vi "RecallState.vi"(8 "error in":errorcluster, 10 "File Name ()":string, 11 "C4209 PNA.lvclass 2":refnum<class "C4209 PNA.lvclass">) -> (0 "error out":errorcluster, 3 "C4209 PNA.lvclass":refnum<class "C4209 PNA.lvclass">)   [LabVIEW 2019, in "C4209 PNA.lvclass"]
uses:
  C4209 PNA.lvclass
  C4209 PNA.lvclass/C4209 PNA.ctl
  <instrlib>/CMT S2 Series VNA/CMT S2 Series VNA.lvlib
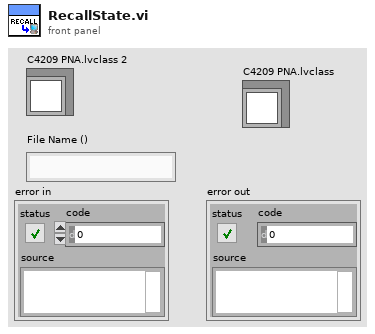
[diagram p1: front panel]
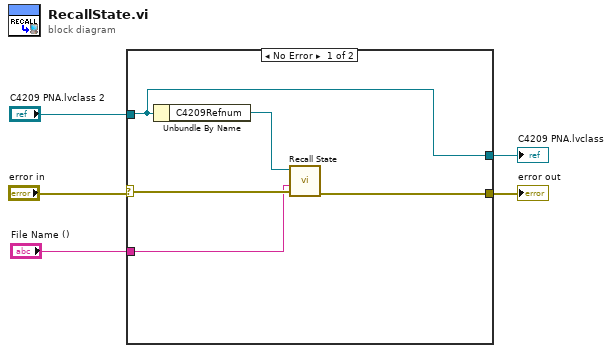
[diagram p0: block diagram]
diagram:
  n1 = case shown="No Error" "error in" {
    selector: "error in" -> [w10 w12]
    tunnel: "C4209 PNA.lvclass 2" -> [w6 w11]
    tunnel: "File Name ()" -> [w8 _]
    tunnel: [w7 w12] -> w1
    tunnel: [w6 w11] -> w2
    frame No Error {
      n2 = Unbundle By Name(w6) -> ("C4209Refnum"=w9:refnum<k7>)
      n3 = call <instrlib>:"Recall State.vi"("error in (no error)"=w10, "File Name ()"=w8, "Reference in"=w9) -> ("error out"=w7:errorcluster)  [unwired: 7 in, 1 out]
    }
    frame Error {
    }
  }
  "C4209 PNA.lvclass" <- w2
  "error out" <- w1
